vi "TDS Digital Input Read.vi"(8 "error in (no error)":errorcluster, 10 "Signal InstConfig":string, 11 "Address":string) -> (0 "error out":errorcluster, 3 "Input State":bool)   [LabVIEW 2025, in "Interface Functions.lvlib"]
uses:
  Interface Functions.lvlib
panel:
  # "Digital Input Read"
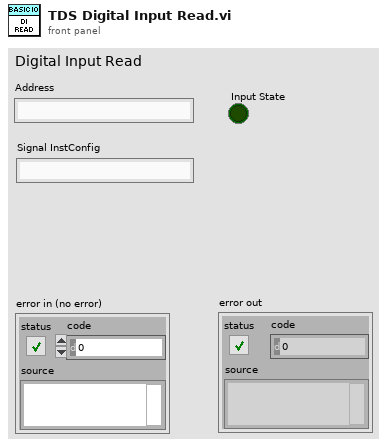
[diagram p1: front panel]
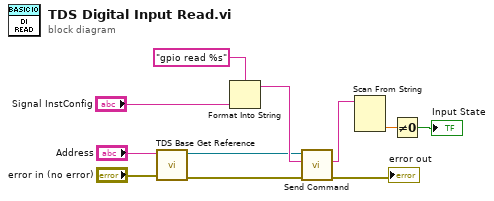
[diagram p0: block diagram]
diagram:
  n1 = call "TDS Base Get Reference.vi"("error in (no error)"="error in (no error)", "Address"="Address") -> ("error out"=w5:errorcluster, "Reference"=w6:refnum<visa-resource-name>)  [unwired: 8 in]
  n2 = Format Into String(format string="gpio read %s", "Signal InstConfig") -> (resulting string=w7:string)  [unwired: 2 in, 1 out]
  n3 = call "Send Command.vi"("error in (no error)"=w5, "Command"=w7, "VISA resource name"=w6) -> ("error out"=→"error out":errorcluster, "Read Value"=w3:string)  [unwired: 6 in, 1 out]
  n4 = Scan From String(input string=w3) -> (output 1=w1:dbl)  [unwired: 4 in, 3 out]
  n5 = Not Equal To 0?(x=w1) -> (x != 0?=→"Input State":bool)
